vi "launcher.vi"() -> ()   [LabVIEW 2013]
panel:
  in  "Stop Button":bool=TRUE
  in  "sg":bool caption="multimeter"
  in  "pg":bool caption="multimeter"
  in  "osci":bool caption="multimeter"
  in  "multimeter":bool
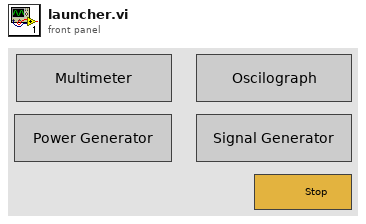
[diagram p1: front panel]
types:
  T1 = enum32{"Invalid", "Standard", "Closed", "Hidden", "Minimized", "Maximized"}
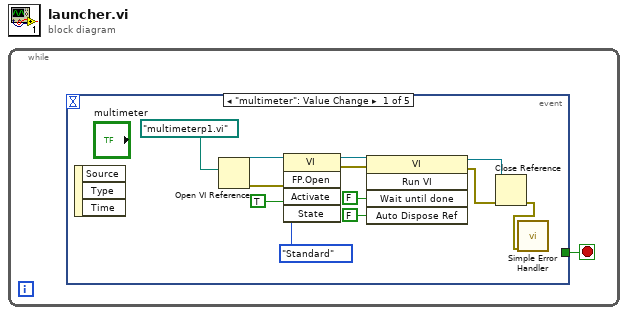
[diagram p0: block diagram]
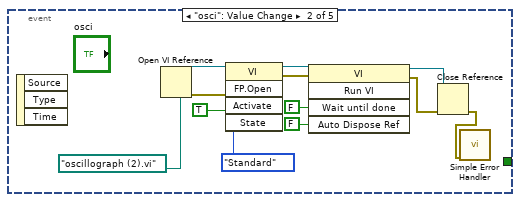
[diagram p2: hidden frame]
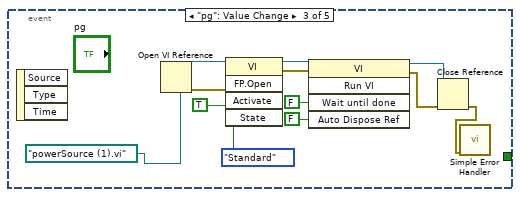
[diagram p3: hidden frame]
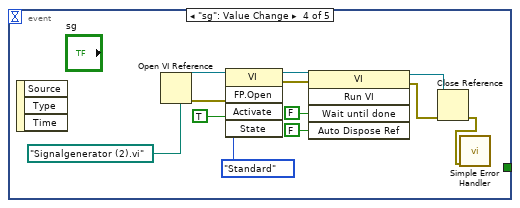
[diagram p4: hidden frame]
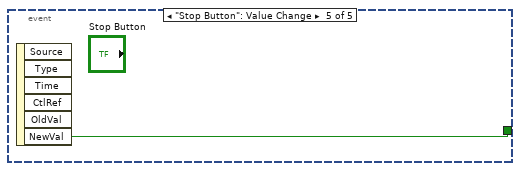
[diagram p5: hidden frame]
diagram:
  n1 = while {
    stop <- w1 stop-if-true
    n2 = event shown="[0] \"multimeter\": Value Change" {
      selector: _ -> [_ _ _ _ _]
      dyn-events: _ -> [_ _ _ _ _]
      timeout: _ -> [_ _ _ _ _]
      tunnel: [_ _ _ _ w50] -> w1
      event "multimeter": Value Change {
        n3 = event-data() -> ()  [unwired: 1 in, 3 out]
        n4 = Open VI Reference(vi path=path "multimeterp1.vi") -> (vi reference=w12:refnum<vi>, error out=w11:errorcluster)  [unwired: 5 in]
        n5 = invoke class="VI" method="FP.Open"(reference=w12, error in=w11, "Activate"=TRUE ("Activate?"), "State"=T1."Standard") -> (reference out=w8:refnum<vi>, error out=w7:errorcluster)  [unwired: 1 in, 3 out]
        n6 = invoke class="VI" method="Run VI"(reference=w8, error in=w7, "Wait until done"=FALSE ("Wait Until Done"), "Auto Dispose Ref"=FALSE ("Auto Dispose Reference")) -> (reference out=w6:refnum<vi>, error out=w5:errorcluster)  [unwired: 1 in, 3 out]
        n7 = Close Reference(reference=w6, error in (no error)=w5) -> (error out=w2:errorcluster)
        n8 = call <vilib>:"Simple Error Handler.vi"("error in (no error)"=w2) -> ()  [unwired: 4 in, 5 out]
      }
      event "osci": Value Change {
        n9 = event-data() -> ()  [unwired: 1 in, 3 out]
        n10 = Open VI Reference(vi path=path "oscillograph (2).vi") -> (vi reference=w25:refnum<vi>, error out=w24:errorcluster)  [unwired: 5 in]
        n11 = invoke class="VI" method="FP.Open"(reference=w25, error in=w24, "Activate"=TRUE ("Activate?"), "State"=T1."Standard") -> (reference out=w21:refnum<vi>, error out=w20:errorcluster)  [unwired: 1 in, 3 out]
        n12 = invoke class="VI" method="Run VI"(reference=w21, error in=w20, "Wait until done"=FALSE ("Wait Until Done"), "Auto Dispose Ref"=FALSE ("Auto Dispose Reference")) -> (reference out=w19:refnum<vi>, error out=w18:errorcluster)  [unwired: 1 in, 3 out]
        n13 = Close Reference(reference=w19, error in (no error)=w18) -> (error out=w15:errorcluster)
        n14 = call <vilib>:"Simple Error Handler.vi"("error in (no error)"=w15) -> ()  [unwired: 4 in, 5 out]
      }
      event "pg": Value Change {
        n15 = event-data() -> ()  [unwired: 1 in, 3 out]
        n16 = Open VI Reference(vi path=path "powerSource (1).vi") -> (vi reference=w37:refnum<vi>, error out=w36:errorcluster)  [unwired: 5 in]
        n17 = invoke class="VI" method="FP.Open"(reference=w37, error in=w36, "Activate"=TRUE ("Activate?"), "State"=T1."Standard") -> (reference out=w33:refnum<vi>, error out=w32:errorcluster)  [unwired: 1 in, 3 out]
        n18 = invoke class="VI" method="Run VI"(reference=w33, error in=w32, "Wait until done"=FALSE ("Wait Until Done"), "Auto Dispose Ref"=FALSE ("Auto Dispose Reference")) -> (reference out=w31:refnum<vi>, error out=w30:errorcluster)  [unwired: 1 in, 3 out]
        n19 = Close Reference(reference=w31, error in (no error)=w30) -> (error out=w27:errorcluster)
        n20 = call <vilib>:"Simple Error Handler.vi"("error in (no error)"=w27) -> ()  [unwired: 4 in, 5 out]
      }
      event "sg": Value Change {
        n21 = event-data() -> ()  [unwired: 1 in, 3 out]
        n22 = Open VI Reference(vi path=path "Signalgenerator (2).vi") -> (vi reference=w49:refnum<vi>, error out=w48:errorcluster)  [unwired: 5 in]
        n23 = invoke class="VI" method="FP.Open"(reference=w49, error in=w48, "Activate"=TRUE ("Activate?"), "State"=T1."Standard") -> (reference out=w45:refnum<vi>, error out=w44:errorcluster)  [unwired: 1 in, 3 out]
        n24 = invoke class="VI" method="Run VI"(reference=w45, error in=w44, "Wait until done"=FALSE ("Wait Until Done"), "Auto Dispose Ref"=FALSE ("Auto Dispose Reference")) -> (reference out=w43:refnum<vi>, error out=w42:errorcluster)  [unwired: 1 in, 3 out]
        n25 = Close Reference(reference=w43, error in (no error)=w42) -> (error out=w39:errorcluster)
        n26 = call <vilib>:"Simple Error Handler.vi"("error in (no error)"=w39) -> ()  [unwired: 4 in, 5 out]
      }
      event "Stop Button": Value Change {
        n27 = event-data() -> ("NewVal"=w50:bool)  [unwired: 1 in, 5 out]
      }
    }
  }
